vi "Load Config.vi"(6 "Constants":refnum<class "Sequence Constants.lvclass">, 8 "error in (no error)":refnum<class "MultiErrors.lvclass">, 10 "Config Element":refnum<class "Config Element.lvclass">, 11 "Condition Config in":refnum<class "Condition Config.lvclass">) -> (0 "error out":refnum<class "MultiErrors.lvclass">, 3 "Condition Config out":refnum<class "Condition Config.lvclass">)   [LabVIEW 2020, in "VolatusSeqConfig.lvlib" / "Condition Config.lvclass"]
uses:
  Condition Config.lvclass
  VolatusErrorUtilities/MultiErrors/MultiErrors.lvclass
  lv-cdm/CDM-Config/Config Element/Config Element.lvclass
  Condition Config.lvclass/Condition Config.ctl
  Sequence Constants/Sequence Constants.lvclass
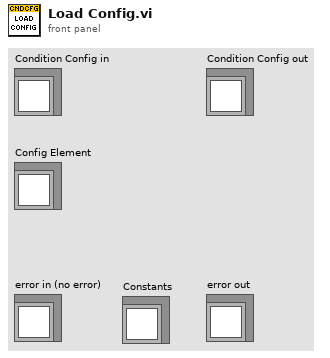
[diagram p1: front panel]
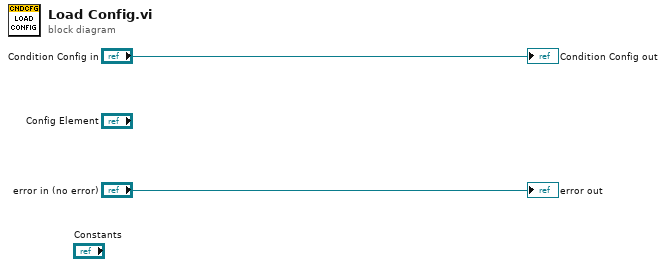
[diagram p0: block diagram]
diagram:
  "error out" <- "error in (no error)"
  "Condition Config out" <- "Condition Config in"
